vi "BNO055 make gyro stop .vi"(8 "error in (no error)":errorcluster) -> (0 "error out":errorcluster)   [LabVIEW 2019]
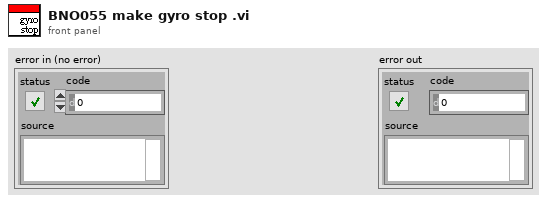
[diagram p1: front panel]
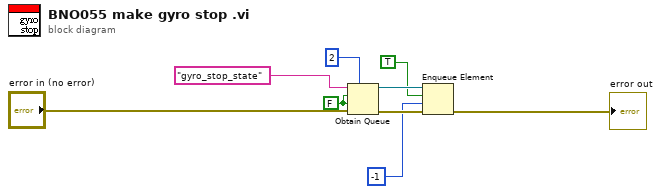
[diagram p0: block diagram]
diagram:
  w1 = FALSE ("create if not found? (T)")
  n1 = Obtain Queue(max queue size (-1, unlimited)=2, name (unnamed)="gyro_stop_state", element data type=w1, create if not found? (T)=w1, error in (no error)="error in (no error)") -> (queue out=w5:refnum<queue>, error out=w6:errorcluster)  [unwired: 1 out]
  n2 = Enqueue Element(queue=w5, element=TRUE, timeout in ms (-1)=-1, error in (no error)=w6) -> (error out=→"error out":errorcluster)  [unwired: 2 out]
